vi "Begin.vi"() -> (0 "error out":errorcluster)   [LabVIEW 2013]
doc: "Called before other user functions, this VI is expected to open initial I/O refnums, load in file data, and do all program initialization. Notice that the <B>error out</B> terminal is simply used for data flow. Wiring it to other structures or subVIs ensures that this VI runs first."
uses:
  <vilib>/Rock Robotics/SystemInterfaces/DIO/FPGA_DIOPWMChannel.ctl
  <vilib>/Rock Robotics/WPI/DriverStation/WPI_DriverStationRobotMode2.ctl
  <vilib>/Rock Robotics/WPI/Joystick/WPI_JoystickDeviceEnum.ctl
  <vilib>/Rock Robotics/WPI/SafetyOutput/WPI_SafetyOutputConfigMenu.ctl
  <vilib>/Rock Robotics/SystemInterfaces/DIO/FPGA_DIOChannel.ctl
  <vilib>/Rock Robotics/WPI/RobotDrive/WPI_RobotDriveOpen2MotorWithJaguar.vi
  Robot Global Data.vi
  <vilib>/Rock Robotics/WPI/MotorControl/WPI_MotorControlOpen Victor.vi
  <vilib>/Rock Robotics/WPI/MotorControl/WPI_MotorControlOpen Talon.vi
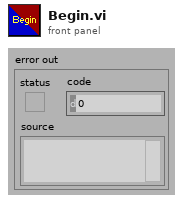
[diagram p1: front panel]
types:
  T1 = typedef "WPI_SafetyOutputConfigMenu.ctl" = enum16{"Enable", "Disable"}
  T2 = typedef "FPGA_DIOPWMChannel.ctl" = enum8{"PWM 1", "PWM 2", "PWM 3", "PWM 4", "PWM 5", "PWM 6", "PWM 7", "PWM 8", "PWM 9", "PWM 10", "Invalid"}
  T3 = typedef "FPGA_DIOChannel.ctl" = enum8{"DIO 1", "DIO 2", "DIO 3", "DIO 4", "DIO 5", "DIO 6", "DIO 7", "DIO 8", "DIO 9", "DIO 10", "DIO 11", "DIO 12", "DIO 13", "DIO 14", "Invalid"}
  T4 = typedef "WPI_JoystickDeviceEnum.ctl" = enum16{"USB 1", "USB 2", "USB 3", "USB 4", "Kinect 1", "Kinect 2"}
  T5 = typedef "WPI_DriverStationRobotMode2.ctl" = enum16{"Autonomous Disabled", "Autonomous Enabled", "Teleop Disabled", "Teleop Enabled", "Timeout", "Finish", "Test Disabled", "Test Enabled"}
  T6 = typedef "WPI_JoystickDevRef.ctl" = cluster{"Device":T4}
  T7 = typedef "WPI_RobotDriveDevRef.ctl" = cluster{"DevStatus":errorcluster, "Motors[]":T8[], "Square Inputs":bool, "Max Output":dbl, "Isochronous":bool}
  T8 = typedef "WPI_MotorControlDeviceRef.ctl" = cluster{"DeviceStatus":errorcluster, "Type":enum16{"PWM", "CAN"}, "PWM":cluster{"Digital Module":T9, "PWM Channel":T2, "DeadBand":T10}, "CAN":cluster{"Device Number":u8, "Control Mode":T11, "Semaphore":T12, "Max Vout":dbl}, "Invert":bool, "TransformRef":T13, "InvTransformRef":T13}
  T9 = typedef "FPGA_TypedefDigitalModule.ctl" = enum16{"Digital Module 1", "Digital Module 2"}
  T10 = typedef "WPI_PWMDeadband.ctl" = cluster{"Name":string, "maxPositivePwm":i32, "minPositivePwm":i32, "centerPwm":i32, "maxNegativePwm":i32, "minNegativePwm":i32, "angularRange":u16}
  T11 = typedef "WPI_CANJaguar_ControlMode.ctl" = enum8{"Percent VBus", "Current", "Speed", "Position", "Voltage"}
  T12 = typedef "Semaphore RefNum" = refnum<k1>
  T13 = typedef "WPI_PWMTransform_ConPane.ctl" = refnum<vi>
  T14 = typedef "WPI_DigitalInputDevRef.ctl" = cluster{"DevStatus":errorcluster, "DIO Channel":T3, "Digital Module":T9}
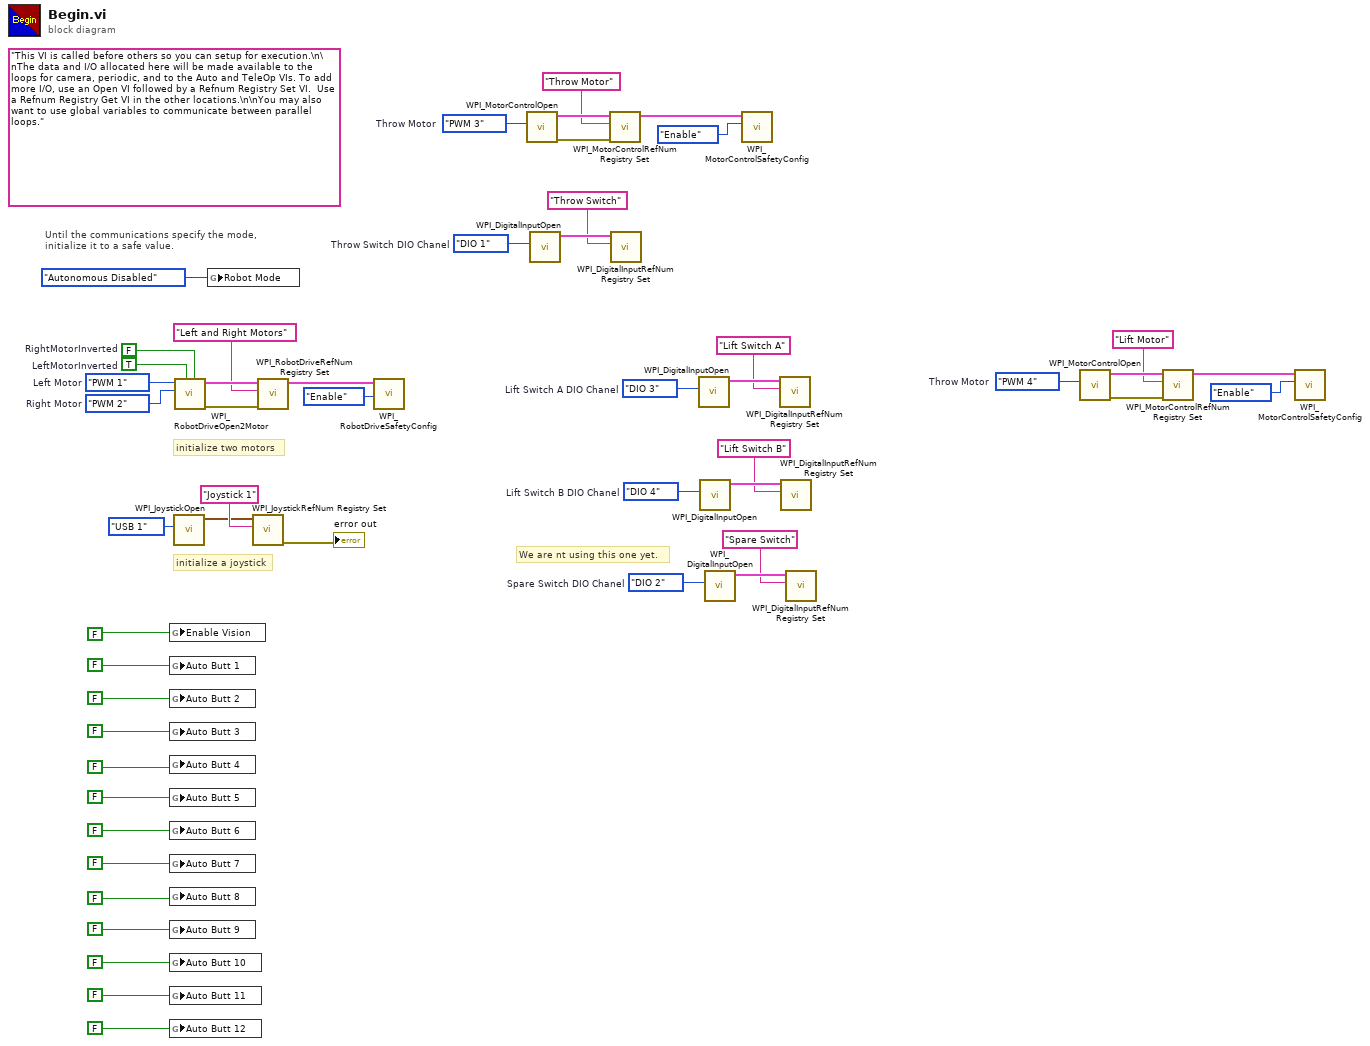
[diagram p0: block diagram]
diagram:
  w17 = FPGA_DIOPWMChannel."PWM 4"  # Throw Motor
  w21 = FPGA_DIOChannel."DIO 2"  # Spare Switch DIO Chanel
  w24 = FPGA_DIOChannel."DIO 4"  # Lift Switch B DIO Chanel
  w27 = FPGA_DIOChannel."DIO 3"  # Lift Switch A DIO Chanel
  w30 = FPGA_DIOChannel."DIO 1"  # Throw Switch DIO Chanel
  w35 = FPGA_DIOPWMChannel."PWM 3"  # Throw Motor
  (unwired) "This VI is called before others so you can setup for execution.\n\nThe data and I/O allocated here will be made available to the loops for camera, periodic, and to the Auto and TeleOp VIs. To add more I/O, use an Open VI followed by a Refnum Registry Set VI.  Use a Refnum Registry Get VI in the other locations.\n\nYou may also want to use global variables to communicate between parallel loops."
  w44 = FPGA_DIOPWMChannel."PWM 2"  # Right Motor
  w45 = FPGA_DIOPWMChannel."PWM 1"  # Left Motor
  w49 = TRUE  # LeftMotorInverted
  w50 = FALSE  # RightMotorInverted
  # "We are nt using this one yet."
  # "initialize a joystick"
  # "Until the communications specify the mode,\ninitialize it to a safe value."
  # "initialize two motors"
  n1 = global write "Robot Global Data.vi" "Enable Vision"(FALSE) -> ()
  n2 = global write "Robot Global Data.vi" "Auto Butt 1"(FALSE) -> ()
  n3 = global write "Robot Global Data.vi" "Auto Butt 2"(FALSE) -> ()
  n4 = global write "Robot Global Data.vi" "Auto Butt 3"(FALSE) -> ()
  n5 = global write "Robot Global Data.vi" "Auto Butt 4"(FALSE) -> ()
  n6 = global write "Robot Global Data.vi" "Auto Butt 5"(FALSE) -> ()
  n7 = global write "Robot Global Data.vi" "Auto Butt 6"(FALSE) -> ()
  n8 = global write "Robot Global Data.vi" "Auto Butt 7"(FALSE) -> ()
  n9 = global write "Robot Global Data.vi" "Auto Butt 8"(FALSE) -> ()
  n10 = global write "Robot Global Data.vi" "Auto Butt 9"(FALSE) -> ()
  n11 = global write "Robot Global Data.vi" "Auto Butt 10"(FALSE) -> ()
  n12 = global write "Robot Global Data.vi" "Auto Butt 11"(FALSE) -> ()
  n13 = global write "Robot Global Data.vi" "Auto Butt 12"(FALSE) -> ()
  n14 = call <vilib>:"WPI_JoystickOpen.vi"("JoystickDevice"=WPI_JoystickDeviceEnum."USB 1") -> ("JoystickDevRef"=w39:T6)  [unwired: 10 in]
  n15 = call-poly <vilib>:"WPI_RobotDriveOpen2Motor.vi"("Right Motor Inverted"=w50, "Left Motor Inverted"=w49, "Right Motor"=w44, "Left Motor"=w45) -> ("error out"=w46:errorcluster, "RobotDriveDevRef"=w48:T7)  [unwired: 1 in, 5 out]
  n16 = global write "Robot Global Data.vi" "Robot Mode"(WPI_DriverStationRobotMode2."Autonomous Disabled" ("Robot Mode")) -> ()
  n17 = call <vilib>:"WPI_JoystickRefNum Registry Set.vi"("refnum name"="Joystick 1", "JoystickDevRef"=w39) -> ("error out"=→"error out":errorcluster)  [unwired: 8 in, 1 out]
  n18 = call <vilib>:"WPI_RobotDriveRefNum Registry Set.vi"("error in (no error)"=w46, "refnum name"="Left and Right Motors", "RobotDriveDevRef"=w48) -> ("RobotDriveDevRef"=w43:T7)  [unwired: 8 out]
  n19 = call <vilib>:"WPI_RobotDriveSafetyConfig.vi"("mode"=WPI_SafetyOutputConfigMenu."Enable", "RobotDriveDevRef"=w43) -> ()  [unwired: 8 in, 2 out]
  n20 = call-poly <vilib>:"WPI_MotorControlOpen.vi"("PWM Channel"=w35) -> ("error out"=w33:errorcluster, "MotorControlDeviceRef"=w51:T8)  [unwired: 6 in, 3 out]
  n21 = call <vilib>:"WPI_DigitalInputOpen.vi"("DIO Channel"=w30) -> ("DigitalInputDevRef"=w29:T14)  [unwired: 9 in, 1 out]
  n22 = call <vilib>:"WPI_MotorControlRefNum Registry Set.vi"("error in (no error)"=w33, "refnum name"="Throw Motor", "MotorControlDevRef"=w51) -> ("MotorControlDevRef"=w32:T8)  [unwired: 7 in, 1 out]
  n23 = call <vilib>:"WPI_DigitalInputRefNum Registry Set.vi"("refnum name"="Throw Switch", "DigitalInputDevRef"=w29) -> ()  [unwired: 8 in, 2 out]
  n24 = call <vilib>:"WPI_DigitalInputOpen.vi"("DIO Channel"=w27) -> ("DigitalInputDevRef"=w26:T14)  [unwired: 9 in, 1 out]
  n25 = call <vilib>:"WPI_DigitalInputOpen.vi"("DIO Channel"=w24) -> ("DigitalInputDevRef"=w23:T14)  [unwired: 9 in, 1 out]
  n26 = call <vilib>:"WPI_DigitalInputOpen.vi"("DIO Channel"=w21) -> ("DigitalInputDevRef"=w20:T14)  [unwired: 9 in, 1 out]
  n27 = call <vilib>:"WPI_MotorControlSafetyConfig.vi"("mode"=WPI_SafetyOutputConfigMenu."Enable", "MotorControlDevRef"=w32) -> ()  [unwired: 8 in, 2 out]
  n28 = call <vilib>:"WPI_DigitalInputRefNum Registry Set.vi"("refnum name"="Lift Switch A", "DigitalInputDevRef"=w26) -> ()  [unwired: 8 in, 2 out]
  n29 = call <vilib>:"WPI_DigitalInputRefNum Registry Set.vi"("refnum name"="Lift Switch B", "DigitalInputDevRef"=w23) -> ()  [unwired: 8 in, 2 out]
  n30 = call <vilib>:"WPI_DigitalInputRefNum Registry Set.vi"("refnum name"="Spare Switch", "DigitalInputDevRef"=w20) -> ()  [unwired: 8 in, 2 out]
  n31 = call-poly <vilib>:"WPI_MotorControlOpen.vi"("PWM Channel"=w17) -> ("error out"=w15:errorcluster, "MotorControlDeviceRef"=w18:T8)  [unwired: 6 in, 3 out]
  n32 = call <vilib>:"WPI_MotorControlRefNum Registry Set.vi"("error in (no error)"=w15, "refnum name"="Lift Motor", "MotorControlDevRef"=w18) -> ("MotorControlDevRef"=w14:T8)  [unwired: 7 in, 1 out]
  n33 = call <vilib>:"WPI_MotorControlSafetyConfig.vi"("mode"=WPI_SafetyOutputConfigMenu."Enable", "MotorControlDevRef"=w14) -> ()  [unwired: 8 in, 2 out]
